vi "Counter Demo.vi"() -> ()   [LabVIEW 2024]
panel:
  out "data":dbl format="%0.2f"
  out "error out":errorcluster caption="错误输出"
  in  "stop":bool
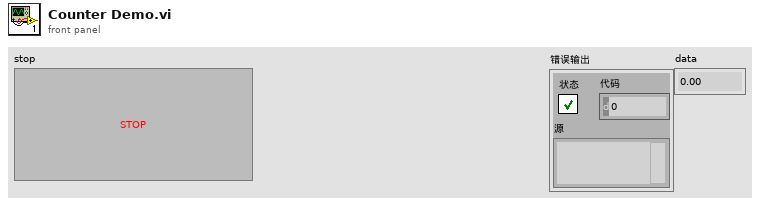
[diagram p1: front panel]
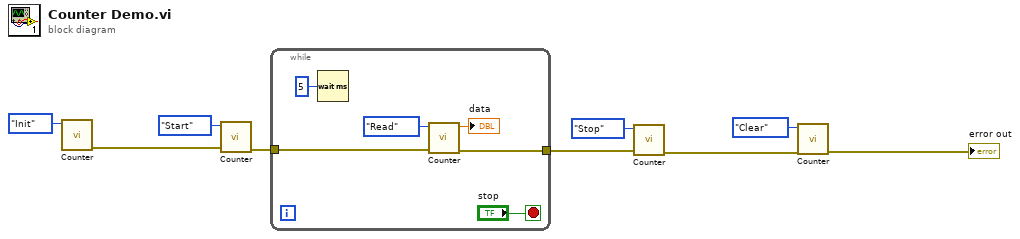
[diagram p0: block diagram]
diagram:
  n1 = call "Counter.vi"("Enum"=enum16{"Init", "Start", "Read", "Stop", "Clear"}."Init") -> ("error out"=w5:errorcluster)  [unwired: 9 in, 1 out]
  n2 = call "Counter.vi"("error in"=w5, "Enum"=enum16{"Init", "Start", "Read", "Stop", "Clear"}."Start") -> ("error out"=w4:errorcluster)  [unwired: 8 in, 1 out]
  n3 = while {
    tunnel: w4 -> [w14]
    tunnel: [w13] -> w3
    stop <- "stop" stop-if-true
    n4 = Wait (ms)(milliseconds to wait=u32 5) -> ()  [unwired: 1 out]
    n5 = call "Counter.vi"("error in"=w14, "Enum"=enum16{"Init", "Start", "Read", "Stop", "Clear"}."Read") -> ("error out"=w13:errorcluster, "data"=→"data":dbl)  [unwired: 8 in]
  }
  n6 = call "Counter.vi"("error in"=w3, "Enum"=enum16{"Init", "Start", "Read", "Stop", "Clear"}."Stop") -> ("error out"=w2:errorcluster)  [unwired: 8 in, 1 out]
  n7 = call "Counter.vi"("error in"=w2, "Enum"=enum16{"Init", "Start", "Read", "Stop", "Clear"}."Clear") -> ("error out"=→"error out":errorcluster)  [unwired: 8 in, 1 out]
